vi "mergeActiveXPropNode.vi"   [LabVIEW 2017]
doc: "Gets (reads) and/or sets (writes) properties of a reference."
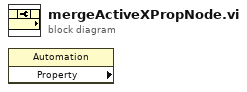
[diagram p0: block diagram]
diagram:
  n1 = property class="Automation" props=[]() -> ()  [unwired: 2 in, 3 out]
